vi "Recall Setup.vi"(8 "Error In (no error)":errorcluster, 9 "Restore Settings (0: None)":u16(ring) items=["None", "Buffer 1", "Buffer 2", "Buffer 3", "Buffer 4", "Buffer 5", "Buffer 6", "Buffer 7", "Buffer 8", "Buffer 9"], 10 "Save Settings (0: None)":u16(ring) items=["None", "Buffer 1", "Buffer 2", "Buffer 3", "Buffer 4", "Buffer 5", "Buffer 6", "Buffer 7", "Buffer 8", "Buffer 9"], 11 "VISA Resource Name":refnum<visa-resource-name>) -> (0 "Error Out":errorcluster, 3 "VISA Resource Name Out":refnum<visa-resource-name>)   [LabVIEW 2010, in "Stanford Research 844.lvlib"]
doc: "This VI saves and recalls instrument's setup."
uses:
  <instrlib>/Stanford Research 844/Stanford Research 844.lvlib
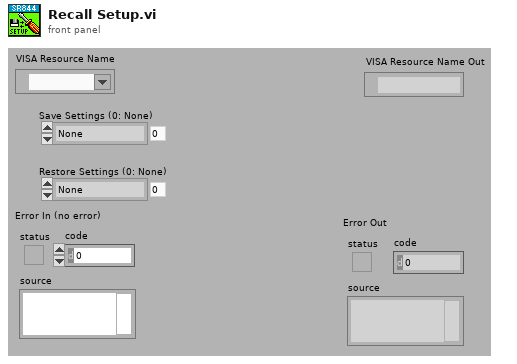
[diagram p1: front panel]
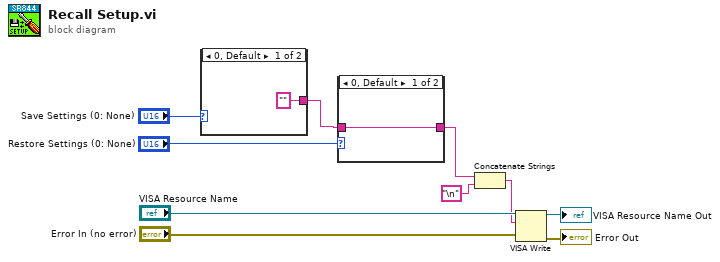
[diagram p0: block diagram]
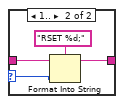
[diagram p2: hidden frame]
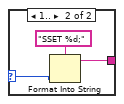
[diagram p3: hidden frame]
diagram:
  n1 = case shown="0, Default" "Save Settings (0: None)" {
    selector: "Save Settings (0: None)" -> [_ w14]
    tunnel: ["" w12] -> w4
    frame 0, Default {
    }
    frame 1.. {
      n2 = Format Into String(format string="SSET %d;", w14) -> (resulting string=w12:string)  [unwired: 2 in, 1 out]
    }
  }
  n3 = case shown="0, Default" "Restore Settings (0: None)" {
    selector: "Restore Settings (0: None)" -> [_ w19]
    tunnel: w4 -> [w15 w17]
    tunnel: [w15 w16] -> w1
    frame 0, Default {
    }
    frame 1.. {
      n4 = Format Into String(format string="RSET %d;", initial string=w17, w19) -> (resulting string=w16:string)  [unwired: 1 in, 1 out]
    }
  }
  n5 = Concatenate Strings(w1, "\n" ("string")) -> (w2:string)
  n6 = VISA Write(VISA resource name="VISA Resource Name", write buffer=w2, error in (no error)="Error In (no error)") -> (VISA resource name out=→"VISA Resource Name Out":refnum<visa-resource-name>, error out=→"Error Out":errorcluster)  [unwired: 1 out]
